vi "Memory.Pointer.Read Bytes.Subset.vi"   [LabVIEW 2016, in "LabVIEW Memory Manager.lvlib" / "Memory.Pointer.lvclass"]
uses:
  Memory.Pointer.lvclass
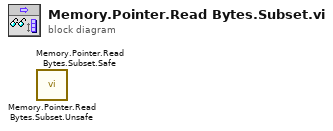
[diagram p0: block diagram]
diagram:
  n1 = call "Memory.Pointer.Read Bytes.Subset.Unsafe.vi"() -> ()  [unwired: 8 in, 4 out]
  n2 = call "Memory.Pointer.Read Bytes.Subset.Safe.vi"() -> ()  [unwired: 8 in, 4 out]
